vi "ResetMissionArrays.vi"(10 "Mission Array Replacement":refnum<class "GenericMission.lvclass">[](array[class]), 11 "Mission Arrays":T1 {"Readable Missions"."Points of Interest"."North" format="%#_10f"; "Readable Missions"."Points of Interest"."East" format="%#_8f"}) -> (3 "Mission Arrays":T1 {"Readable Missions"."Points of Interest"."North" format="%#_10f"; "Readable Missions"."Points of Interest"."East" format="%#_8f"})   [LabVIEW 2013]
doc: "This VI takes in a given mission array and resets the OCU array cluster using that mission array. This is used for taking the missions from Main and resetting the OCU missions with them. It is useful when Main has been running for a while and already has missions, and you need to restart the OCU.\n\nEric Schneider, August 2014"
uses:
  TypeDef/mission_arrays.ctl
  cRIO_Code/Data/TypeDefs/MissionDescription.ctl
  cRIO_Code/Data/TypeDefs/MissionTypeControl.ctl
  cRIO_Code/Data/TypeDefs/UTM Location.ctl
  cRIO_Code/Logic/Classes/Missions/GenericMission/GenericMission.lvclass
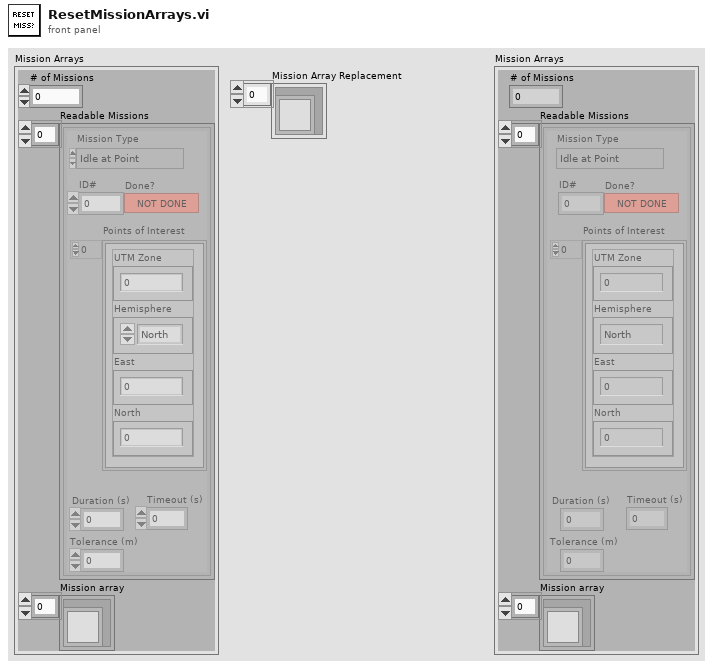
[diagram p1: front panel]
types:
  T1 = typedef "mission_arrays.ctl" = cluster{"# of Missions":i32, "Readable Missions":T2[], "Mission array":refnum<class "GenericMission.lvclass">[]}
  T2 = typedef "MissionDescription.ctl" = cluster{"Duration (s)":dbl, "Timeout (s)":dbl, "Tolerance (m)":dbl, "Mission Type":T3, "Points of Interest":T4[], "ID#":i32, "Done?":bool}
  T3 = typedef "MissionTypeControl.ctl" = enum16{"Idle at Point", "Drive to Waypoint", "Round Buoy to Port", "Round Buoy to Starboard", "Pass Between Buoys", "Station Keeping"}
  T4 = typedef "UTM Location.ctl" = cluster{"UTM Zone":dbl, "Hemisphere":enum16{"North", "South"}, "East":dbl, "North":dbl}
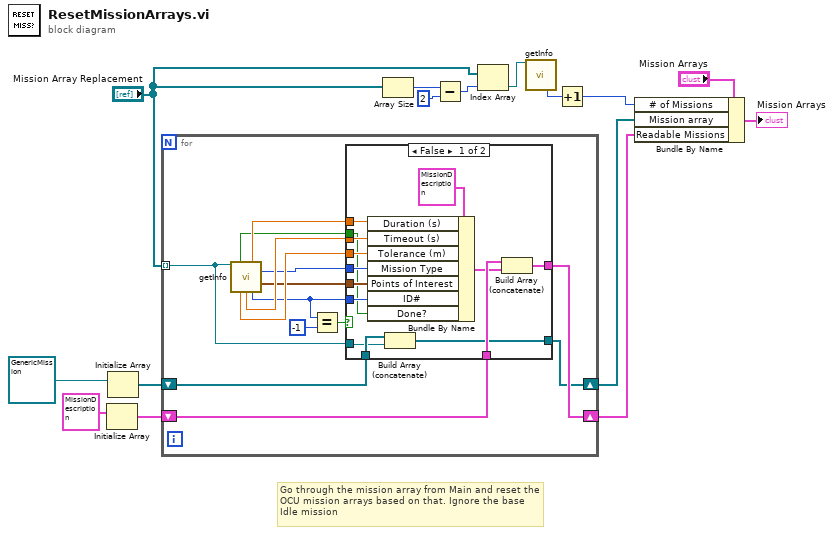
[diagram p0: block diagram]
diagram:
  # "Go through the mission array from Main and reset the OCU mission arrays based on that. Ignore the base Idle mission"
  n1 = Initialize Array(T2 {"Duration (s)"=-1.0, "Timeout (s)"=-1.0, "Tolerance (m)"=0.0, "Mission Type"=enum."Idle at Point", "Points of Interest"=[], "ID#"=0, "Done?"=FALSE} ("element")) -> (w5:T2[])  [unwired: 1 in]
  n2 = Initialize Array(refnum<class "GenericMission.lvclass"> refnum ("GenericMission.lvclass")) -> (w2:refnum<class "GenericMission.lvclass">[])  [unwired: 1 in]
  n3 = for {
    tunnel: "Mission Array Replacement" -> [w17] mode=indexing
    shift-right: [w19] -> w4
    shift-left: w5 -> [w20]
    shift-right: [w16] -> w1
    shift-left: w2 -> [w18]
    n4 = call-dynamic "getInfo.vi"("GenericMission in"=w17) -> ("Done"=w24:bool, "Duration (s)"=w29:dbl, "Mission Type"=w26:T3, "Points of Interest"=w25:T4[], "Tolerance (m)"=w28:dbl, "Timeout (s)"=w27:dbl, "ID#"=w22:i16)  [unwired: 6 in, 2 out]
    n5 = Equal?(x=w22, y=i16 -1) -> (x = y?=w23:bool)
    n6 = case shown="False" w23 {
      tunnel: w29 -> [w42 _]
      tunnel: w28 -> [w41 _]
      tunnel: w27 -> [w40 _]
      tunnel: w26 -> [w39 _]
      tunnel: w25 -> [w38 _]
      tunnel: w22 -> [w37 _]
      tunnel: w24 -> [w36 _]
      tunnel: [w35 w45] -> w19
      tunnel: w20 -> [w34 w45]
      tunnel: w18 -> [w32 w44]
      tunnel: w17 -> [w31 _]
      tunnel: [w30 w44] -> w16
      frame False {
        n7 = Bundle By Name(cluster=T2 {"Duration (s)"=-1.0, "Timeout (s)"=-1.0, "Tolerance (m)"=0.0, "Mission Type"=enum."Idle at Point", "Points of Interest"=[], "ID#"=0, "Done?"=FALSE} ("element"), "Duration (s)"=w42, "Timeout (s)"=w40, "Tolerance (m)"=w41, "Mission Type"=w39, "Points of Interest"=w38, "ID#"=w37, "Done?"=w36) -> (w33:T2)
        n8 = Build Array (concatenate)(w32, w31) -> (w30:refnum<class "GenericMission.lvclass">[])
        n9 = Build Array (concatenate)(w34, w33) -> (w35:T2[])
      }
      frame True {
      }
    }
  }
  n10 = Array Size(array="Mission Array Replacement") -> (size(s)=w9:i32)
  n11 = Subtract(x=w9, y=2) -> (x-y=w7:i32)
  n12 = Index Array(array="Mission Array Replacement", index=w7) -> (element=w13:refnum<class "GenericMission.lvclass">)
  n13 = call-dynamic "getInfo.vi"("GenericMission in"=w13) -> ("ID#"=w12:i16)  [unwired: 6 in, 8 out]
  n14 = Increment(x=w12) -> (x+1=w11:i16)
  n15 = Bundle By Name(cluster="Mission Arrays", "# of Missions"=w11, "Mission array"=w1, "Readable Missions"=w4) -> (→"Mission Arrays":T1)
